vi "Test Path Not Found Error.vi"() -> ()   [LabVIEW 2021]
uses:
  SubVIs/File Not Found Error Core.vi
  File_CIF_U.lvlib
panel:
  out "error out":errorcluster
  out "Pass":bool
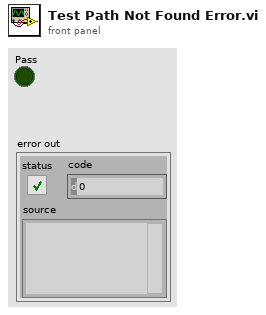
[diagram p1: front panel]
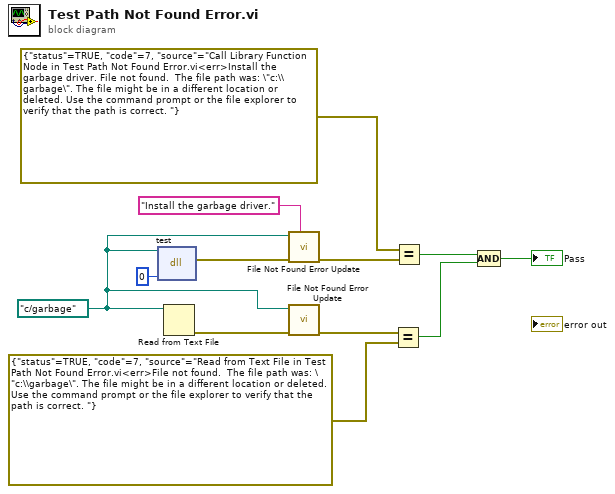
[diagram p0: block diagram]
diagram:
  w8 = path "c:/garbage" ("file (use dialog)")
  n1 = dll-call lib="?" fn="test"(path in=w8, "arg1"=0) -> (error out=w11:errorcluster)  [unwired: 4 in, 1 out]
  n2 = Read from Text File(file (use dialog)=w8) -> (error out=w9:errorcluster)  [unwired: 3 in, 3 out]
  n3 = call "File Not Found Error Update.vi"("Custom Message"="Install the garbage driver.", "error in"=w11, "path in"=w8) -> ("error out"=w5:errorcluster)  [unwired: 8 in]
  n4 = call "File Not Found Error Update.vi"("error in"=w9, "path in"=w8) -> ("error out"=w7:errorcluster)  [unwired: 9 in]
  n5 = Equal?(x=w7, y=errorcluster {"status"=TRUE, "code"=7, "source"="Read from Text File in Test Path Not Found Error.vi<err>File not found.  The file path was: \"c:\\garbage\". The file might be in a different location or deleted. Use the command prompt or the file explorer to verify that the path is correct. "} ("error out 2")) -> (x = y?=w2:bool)
  n6 = Equal?(x=errorcluster {"status"=TRUE, "code"=7, "source"="Call Library Function Node in Test Path Not Found Error.vi<err>Install the garbage driver. File not found.  The file path was: \"c:\\garbage\". The file might be in a different location or deleted. Use the command prompt or the file explorer to verify that the path is correct. "} ("error out"), y=w5) -> (x = y?=w3:bool)
  n7 = Compound Arithmetic op=AND(w3, w2) -> (→"Pass":bool)
